vi "RDS Child Receive Message.vi"(8 "error in (no error)":errorcluster, 10 "RDS Message":refnum<class "RDS Message.lvclass">, 11 "AIP Instrument in":refnum<class "AIP Instrument.lvclass">) -> (0 "error out":errorcluster, 3 "AIP Instrument out":refnum<class "AIP Instrument.lvclass">)   [LabVIEW 2015, in "AIP Instrument.lvlib" / "AIP Instrument.lvclass"]
uses:
  AIP Instrument.lvclass
  Libraries/RDS Framework/RDS Message Class/RDS Message.lvclass
  Libraries/RDS Framework/RDS Message Class/RDS Message.lvclass/RDS Message.ctl
  Libraries/RDS Framework/RDS Message Class/AIP Command.lvclass
  Libraries/RDS Framework/RDS Message Class/AIP Command.lvclass/AIP Command.ctl
  Libraries/RDS Serial Handler/RDS Serial Frame.lvclass/RDS Serial Frame.ctl
  AIP Instrument.lvclass/AIP Instrument.ctl
  Libraries/RDS Child Messages/Depth Data Message/Depth Data Message.lvclass
  Libraries/RDS Instruments/AIP/AIP Status.ctl
  Libraries/RDS Instruments/AIP/AIP States.ctl
  Libraries/RDS Child Messages/Depth Data Message/Depth Data Message.lvclass/Depth Data Message.ctl
  Libraries/RDS Child Messages/AIP Set Min Depth Message/AIP Set Min Depth Message.lvclass
  Libraries/RDS Child Messages/AIP Set Min Depth Message/AIP Set Min Depth Message.lvclass/AIP Set Min Depth Message.ctl
  Libraries/RDS Serial Handler/RDS Serial Frame.lvclass
  Actors/RDS Serial Instrument Actor/RDS Serial Instrument Actor.lvclass
  Libraries/RDS Instruments/RDS Instrument Library.lvlib
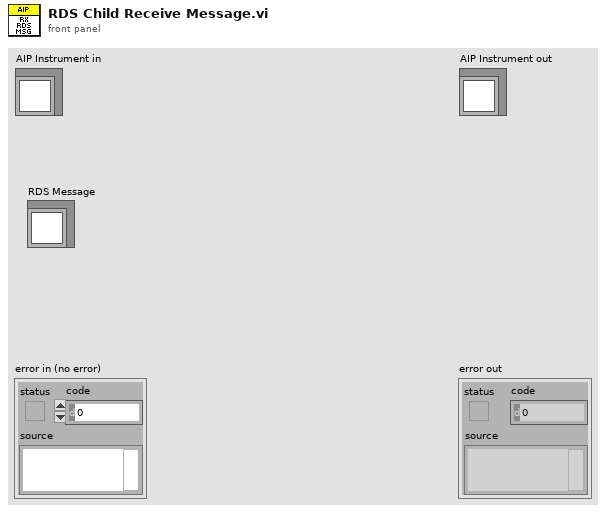
[diagram p1: front panel]
types:
  T1 = typedef "RDS Child Messages.lvlib/RDS Message ID.ctl" = enum16{"RDS Hello World", "String Message", "AIP_Status", "AIP_Command", "GPS_Data", "MCB_Command", "MCB_Status", "Compass_Data", "Depth_Data", "Battery_Data", "Contoller_State", "Set_Mag_Dev", "BTB_Shutdown", "State_Sample_Request", "State_Sample", "PID_Gains_Set", "Helm_Limiter_Set", "Helm_Heading_Command", "Helm_Steering_Command", "Helm_Status", "Controller_Message", "AIP_Set_Min_Depth", "Mission_Controller_State", "Mission_Upload", "Mission_Set_Op_and_Run", "Mission_Settings_Set"}
  T2 = typedef "RDS Instrument Library.lvlib/AIP Status.ctl" = cluster{"FWD Port":T3, "FWD Stbd":T3, "AFT Port":T3, "AFT Stbd":T3, "AIP Depth Min":u8}
  T3 = typedef "RDS Instrument Library.lvlib/AIP States.ctl" = enum16{"Deploy", "Deploying", "Deployed", "Stow", "Stowing", "Stowed", "Fault", "brakeOnStow", "breakOnDeploy", "Stopped", "Stopping"}
  T4 = typedef "RDS Child Messages.lvlib/AIP Command Control.ctl" = enum16{"Stow", "Deploy", "Stop", "Validate Sensors", "Jog Deploy FP", "Jog Stow FP", "Jog Deploy FS", "Jog Stow FS", "Jog Deploy AP", "Jog Stow AP", "Jog Deploy AS", "Jog Stow AS", "Deploy FP", "Deploy FS", "Deploy AP", "Deploy AS", "Stow FP", "Stow FS", "Stow AP", "Stow AS"}
  T5 = typedef "RDS Child Messages.lvlib/Depth Data.ctl" = cluster{"Depth":sgl, "Water Temp":i8}
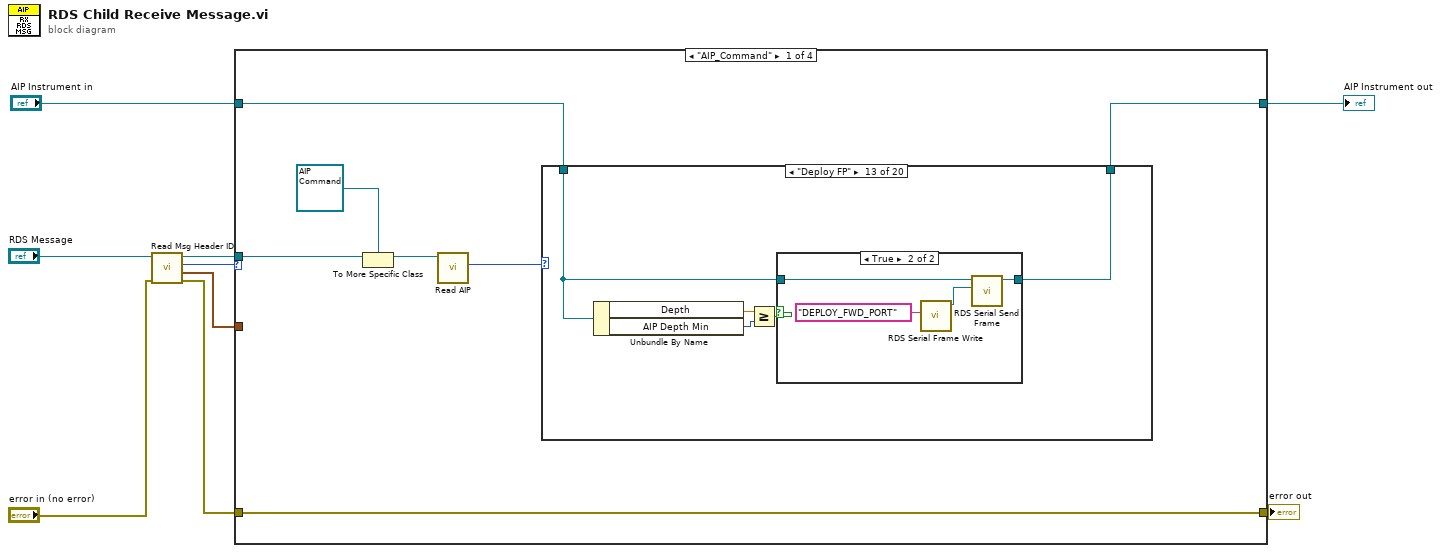
[diagram p0: block diagram]
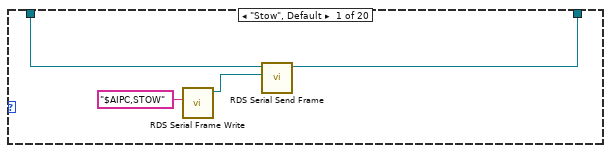
[diagram p2: hidden frame]
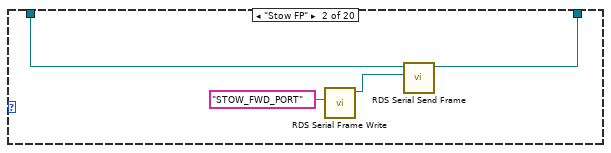
[diagram p3: hidden frame]
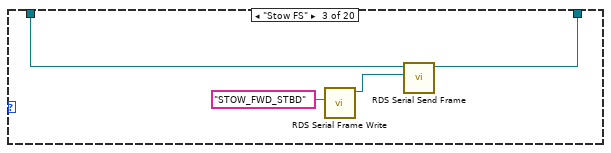
[diagram p4: hidden frame]
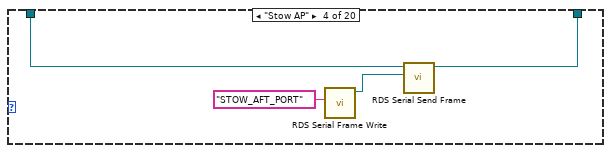
[diagram p5: hidden frame]
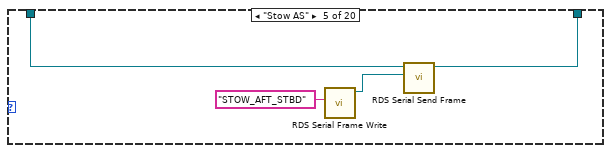
[diagram p6: hidden frame]
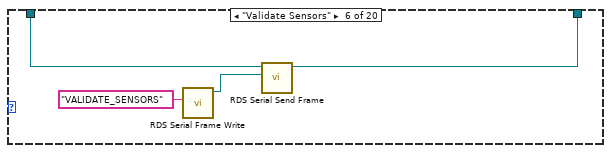
[diagram p7: hidden frame]
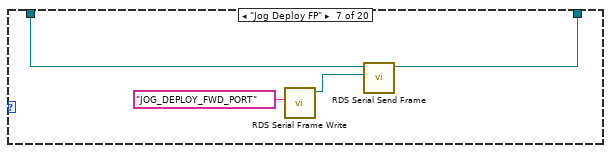
[diagram p8: hidden frame]
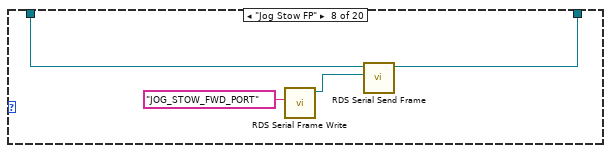
[diagram p9: hidden frame]
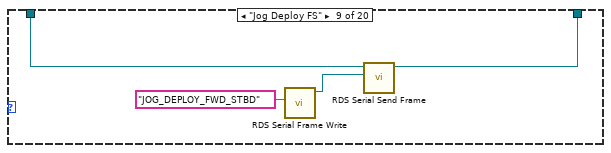
[diagram p10: hidden frame]
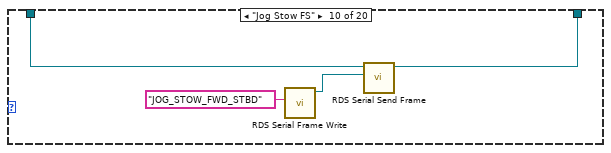
[diagram p11: hidden frame]
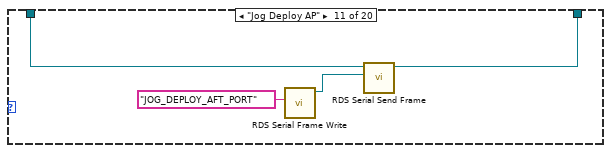
[diagram p12: hidden frame]
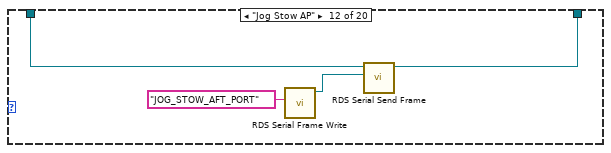
[diagram p13: hidden frame]
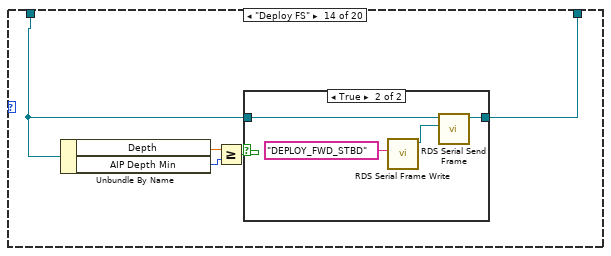
[diagram p15: hidden frame]
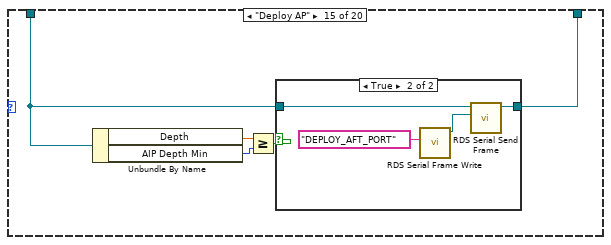
[diagram p17: hidden frame]
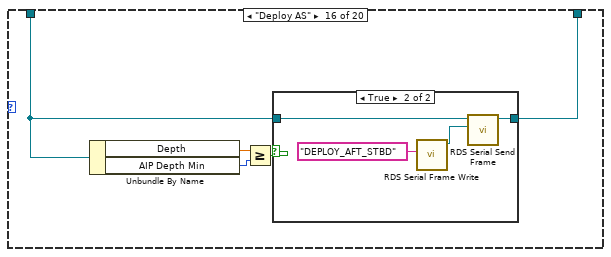
[diagram p19: hidden frame]
diagram:
  n1 = call "Read Msg Header ID.vi"("error in (no error)"="error in (no error)", "RDS Message in"="RDS Message") -> ("error out"=w6:errorcluster, "Time Stamp"=w7:timestamp, "Msg ID"=w9:T1, "RDS Message out"=w8:refnum<class "RDS Message.lvclass">)  [unwired: 5 in, 1 out]
  n2 = case shown="\"AIP_Command\"" w9 {
    tunnel: "AIP Instrument in" -> [w11 w128 w138 w152]
    tunnel: w8 -> [w14 _ w142 w156]
    tunnel: [w10 w128 w129 w151] -> w2
    tunnel: w7 -> [_ _ _ _]
    tunnel: w6 -> [w16 w127 w144 w157]
    tunnel: [w16 w127 w144 w157] -> w1
    frame "AIP_Command" {
      n3 = To More Specific Class(target class=refnum<class "AIP Command.lvclass"> refnum ("RDS Child Messages.lvlib:AIP Command.lvclass"), reference=w14) -> (specific class reference=w13:refnum<class "AIP Command.lvclass">)  [unwired: 1 in, 1 out]
      n4 = call "Read AIP.vi"("AIP Deploy Command in"=w13) -> ("AIP Command"=w12:T4)  [unwired: 8 in, 2 out]
      n5 = case shown="\"Deploy FP\"" w12 {
        tunnel: w11 -> [w18 w22 w26 w30 w34 w38 w42 w46 w50 w54 w58 w62 w66 w76 w86 w95 w106 w110 w116 w126]
        tunnel: [w17 w21 w25 w29 w33 w37 w41 w45 w49 w53 w57 w61 w65 w75 w85 w96 w105 w109 w117 w123] -> w10
        frame "Stow", Default {
          n6 = call "RDS Serial Frame Write.vi"("Serial String"="$AIPC,STOW") -> ("RDS Serial Frame out"=w19:refnum<class "RDS Serial Frame.lvclass">)  [unwired: 9 in, 1 out]
          n7 = call "RDS Serial Send Frame.vi"("RDS Frame"=w19, "RDS Serial Instrument Actor in"=w18) -> ("RDS Serial Instrument Actor out"=w17:refnum<class "AIP Instrument.lvclass">)  [unwired: 8 in, 1 out]
        }
        frame "Stow FP" {
          n8 = call "RDS Serial Frame Write.vi"("Serial String"="STOW_FWD_PORT") -> ("RDS Serial Frame out"=w23:refnum<class "RDS Serial Frame.lvclass">)  [unwired: 9 in, 1 out]
          n9 = call "RDS Serial Send Frame.vi"("RDS Frame"=w23, "RDS Serial Instrument Actor in"=w22) -> ("RDS Serial Instrument Actor out"=w21:refnum<class "AIP Instrument.lvclass">)  [unwired: 8 in, 1 out]
        }
        frame "Stow FS" {
          n10 = call "RDS Serial Frame Write.vi"("Serial String"="STOW_FWD_STBD") -> ("RDS Serial Frame out"=w27:refnum<class "RDS Serial Frame.lvclass">)  [unwired: 9 in, 1 out]
          n11 = call "RDS Serial Send Frame.vi"("RDS Frame"=w27, "RDS Serial Instrument Actor in"=w26) -> ("RDS Serial Instrument Actor out"=w25:refnum<class "AIP Instrument.lvclass">)  [unwired: 8 in, 1 out]
        }
        frame "Stow AP" {
          n12 = call "RDS Serial Frame Write.vi"("Serial String"="STOW_AFT_PORT") -> ("RDS Serial Frame out"=w31:refnum<class "RDS Serial Frame.lvclass">)  [unwired: 9 in, 1 out]
          n13 = call "RDS Serial Send Frame.vi"("RDS Frame"=w31, "RDS Serial Instrument Actor in"=w30) -> ("RDS Serial Instrument Actor out"=w29:refnum<class "AIP Instrument.lvclass">)  [unwired: 8 in, 1 out]
        }
        frame "Stow AS" {
          n14 = call "RDS Serial Frame Write.vi"("Serial String"="STOW_AFT_STBD") -> ("RDS Serial Frame out"=w35:refnum<class "RDS Serial Frame.lvclass">)  [unwired: 9 in, 1 out]
          n15 = call "RDS Serial Send Frame.vi"("RDS Frame"=w35, "RDS Serial Instrument Actor in"=w34) -> ("RDS Serial Instrument Actor out"=w33:refnum<class "AIP Instrument.lvclass">)  [unwired: 8 in, 1 out]
        }
        frame "Validate Sensors" {
          n16 = call "RDS Serial Frame Write.vi"("Serial String"="VALIDATE_SENSORS") -> ("RDS Serial Frame out"=w39:refnum<class "RDS Serial Frame.lvclass">)  [unwired: 9 in, 1 out]
          n17 = call "RDS Serial Send Frame.vi"("RDS Frame"=w39, "RDS Serial Instrument Actor in"=w38) -> ("RDS Serial Instrument Actor out"=w37:refnum<class "AIP Instrument.lvclass">)  [unwired: 8 in, 1 out]
        }
        frame "Jog Deploy FP" {
          n18 = call "RDS Serial Frame Write.vi"("Serial String"="JOG_DEPLOY_FWD_PORT") -> ("RDS Serial Frame out"=w43:refnum<class "RDS Serial Frame.lvclass">)  [unwired: 9 in, 1 out]
          n19 = call "RDS Serial Send Frame.vi"("RDS Frame"=w43, "RDS Serial Instrument Actor in"=w42) -> ("RDS Serial Instrument Actor out"=w41:refnum<class "AIP Instrument.lvclass">)  [unwired: 8 in, 1 out]
        }
        frame "Jog Stow FP" {
          n20 = call "RDS Serial Frame Write.vi"("Serial String"="JOG_STOW_FWD_PORT") -> ("RDS Serial Frame out"=w47:refnum<class "RDS Serial Frame.lvclass">)  [unwired: 9 in, 1 out]
          n21 = call "RDS Serial Send Frame.vi"("RDS Frame"=w47, "RDS Serial Instrument Actor in"=w46) -> ("RDS Serial Instrument Actor out"=w45:refnum<class "AIP Instrument.lvclass">)  [unwired: 8 in, 1 out]
        }
        frame "Jog Deploy FS" {
          n22 = call "RDS Serial Frame Write.vi"("Serial String"="JOG_DEPLOY_FWD_STBD") -> ("RDS Serial Frame out"=w51:refnum<class "RDS Serial Frame.lvclass">)  [unwired: 9 in, 1 out]
          n23 = call "RDS Serial Send Frame.vi"("RDS Frame"=w51, "RDS Serial Instrument Actor in"=w50) -> ("RDS Serial Instrument Actor out"=w49:refnum<class "AIP Instrument.lvclass">)  [unwired: 8 in, 1 out]
        }
        frame "Jog Stow FS" {
          n24 = call "RDS Serial Frame Write.vi"("Serial String"="JOG_STOW_FWD_STBD") -> ("RDS Serial Frame out"=w55:refnum<class "RDS Serial Frame.lvclass">)  [unwired: 9 in, 1 out]
          n25 = call "RDS Serial Send Frame.vi"("RDS Frame"=w55, "RDS Serial Instrument Actor in"=w54) -> ("RDS Serial Instrument Actor out"=w53:refnum<class "AIP Instrument.lvclass">)  [unwired: 8 in, 1 out]
        }
        frame "Jog Deploy AP" {
          n26 = call "RDS Serial Frame Write.vi"("Serial String"="JOG_DEPLOY_AFT_PORT") -> ("RDS Serial Frame out"=w59:refnum<class "RDS Serial Frame.lvclass">)  [unwired: 9 in, 1 out]
          n27 = call "RDS Serial Send Frame.vi"("RDS Frame"=w59, "RDS Serial Instrument Actor in"=w58) -> ("RDS Serial Instrument Actor out"=w57:refnum<class "AIP Instrument.lvclass">)  [unwired: 8 in, 1 out]
        }
        frame "Jog Stow AP" {
          n28 = call "RDS Serial Frame Write.vi"("Serial String"="JOG_STOW_AFT_PORT") -> ("RDS Serial Frame out"=w63:refnum<class "RDS Serial Frame.lvclass">)  [unwired: 9 in, 1 out]
          n29 = call "RDS Serial Send Frame.vi"("RDS Frame"=w63, "RDS Serial Instrument Actor in"=w62) -> ("RDS Serial Instrument Actor out"=w61:refnum<class "AIP Instrument.lvclass">)  [unwired: 8 in, 1 out]
        }
        frame "Deploy FP" {
          n30 = Unbundle By Name(w66) -> ("Depth"=w68:sgl, "AIP Depth Min"=w67:u8)
          n31 = Greater Or Equal?(x=w68, y=w67) -> (x >= y?=w69:bool)
          n32 = case shown="True" w69 {
            tunnel: [w70 w72] -> w65
            tunnel: w66 -> [w70 w71]
            frame False {
              # "TOO SHALLOW!"
            }
            frame True {
              n33 = call "RDS Serial Frame Write.vi"("Serial String"="DEPLOY_FWD_PORT") -> ("RDS Serial Frame out"=w73:refnum<class "RDS Serial Frame.lvclass">)  [unwired: 9 in, 1 out]
              n34 = call "RDS Serial Send Frame.vi"("RDS Frame"=w73, "RDS Serial Instrument Actor in"=w71) -> ("RDS Serial Instrument Actor out"=w72:refnum<class "AIP Instrument.lvclass">)  [unwired: 8 in, 1 out]
            }
          }
        }
        frame "Deploy FS" {
          n35 = Unbundle By Name(w76) -> ("Depth"=w78:sgl, "AIP Depth Min"=w77:u8)
          n36 = Greater Or Equal?(x=w78, y=w77) -> (x >= y?=w79:bool)
          n37 = case shown="True" w79 {
            tunnel: [w80 w82] -> w75
            tunnel: w76 -> [w80 w81]
            frame False {
              # "TOO SHALLOW!"
            }
            frame True {
              n38 = call "RDS Serial Frame Write.vi"("Serial String"="DEPLOY_FWD_STBD") -> ("RDS Serial Frame out"=w83:refnum<class "RDS Serial Frame.lvclass">)  [unwired: 9 in, 1 out]
              n39 = call "RDS Serial Send Frame.vi"("RDS Frame"=w83, "RDS Serial Instrument Actor in"=w81) -> ("RDS Serial Instrument Actor out"=w82:refnum<class "AIP Instrument.lvclass">)  [unwired: 8 in, 1 out]
            }
          }
        }
        frame "Deploy AP" {
          n40 = Unbundle By Name(w86) -> ("Depth"=w88:sgl, "AIP Depth Min"=w87:u8)
          n41 = Greater Or Equal?(x=w88, y=w87) -> (x >= y?=w89:bool)
          n42 = case shown="True" w89 {
            tunnel: [w90 w92] -> w85
            tunnel: w86 -> [w90 w91]
            frame False {
              # "TOO SHALLOW!"
            }
            frame True {
              n43 = call "RDS Serial Frame Write.vi"("Serial String"="DEPLOY_AFT_PORT") -> ("RDS Serial Frame out"=w93:refnum<class "RDS Serial Frame.lvclass">)  [unwired: 9 in, 1 out]
              n44 = call "RDS Serial Send Frame.vi"("RDS Frame"=w93, "RDS Serial Instrument Actor in"=w91) -> ("RDS Serial Instrument Actor out"=w92:refnum<class "AIP Instrument.lvclass">)  [unwired: 8 in, 1 out]
            }
          }
        }
        frame "Deploy AS" {
          n45 = Unbundle By Name(w95) -> ("Depth"=w98:sgl, "AIP Depth Min"=w97:u8)
          n46 = Greater Or Equal?(x=w98, y=w97) -> (x >= y?=w99:bool)
          n47 = case shown="True" w99 {
            tunnel: [w100 w102] -> w96
            tunnel: w95 -> [w100 w101]
            frame False {
              # "TOO SHALLOW!"
            }
            frame True {
              n48 = call "RDS Serial Frame Write.vi"("Serial String"="DEPLOY_AFT_STBD") -> ("RDS Serial Frame out"=w103:refnum<class "RDS Serial Frame.lvclass">)  [unwired: 9 in, 1 out]
              n49 = call "RDS Serial Send Frame.vi"("RDS Frame"=w103, "RDS Serial Instrument Actor in"=w101) -> ("RDS Serial Instrument Actor out"=w102:refnum<class "AIP Instrument.lvclass">)  [unwired: 8 in, 1 out]
            }
          }
        }
        frame "Jog Deploy AS" {
          n50 = call "RDS Serial Frame Write.vi"("Serial String"="JOG_DEPLOY_AFT_STBD") -> ("RDS Serial Frame out"=w107:refnum<class "RDS Serial Frame.lvclass">)  [unwired: 9 in, 1 out]
          n51 = call "RDS Serial Send Frame.vi"("RDS Frame"=w107, "RDS Serial Instrument Actor in"=w106) -> ("RDS Serial Instrument Actor out"=w105:refnum<class "AIP Instrument.lvclass">)  [unwired: 8 in, 1 out]
        }
        frame "Jog Stow AS" {
          n52 = call "RDS Serial Frame Write.vi"("Serial String"="JOG_STOW_AFT_STBD") -> ("RDS Serial Frame out"=w111:refnum<class "RDS Serial Frame.lvclass">)  [unwired: 9 in, 1 out]
          n53 = call "RDS Serial Send Frame.vi"("RDS Frame"=w111, "RDS Serial Instrument Actor in"=w110) -> ("RDS Serial Instrument Actor out"=w109:refnum<class "AIP Instrument.lvclass">)  [unwired: 8 in, 1 out]
        }
        frame "Deploy" {
          n54 = Unbundle By Name(w116) -> ("Depth"=w114:sgl, "AIP Depth Min"=w113:u8)
          n55 = Greater Or Equal?(x=w114, y=w113) -> (x >= y?=w115:bool)
          n56 = case shown="True" w115 {
            tunnel: [w118 w120] -> w117
            tunnel: w116 -> [w118 w119]
            frame False {
              # "TOO SHALLOW!"
            }
            frame True {
              n57 = call "RDS Serial Frame Write.vi"("Serial String"="$AIPC,DEPLOY") -> ("RDS Serial Frame out"=w121:refnum<class "RDS Serial Frame.lvclass">)  [unwired: 9 in, 1 out]
              n58 = call "RDS Serial Send Frame.vi"("RDS Frame"=w121, "RDS Serial Instrument Actor in"=w119) -> ("RDS Serial Instrument Actor out"=w120:refnum<class "AIP Instrument.lvclass">)  [unwired: 8 in, 1 out]
            }
          }
        }
        frame "Stop" {
          n59 = call "RDS Serial Frame Write.vi"("Serial String"="$AIPC,STOP") -> ("RDS Serial Frame out"=w124:refnum<class "RDS Serial Frame.lvclass">)  [unwired: 9 in, 1 out]
          n60 = call "RDS Serial Send Frame.vi"("RDS Frame"=w124, "RDS Serial Instrument Actor in"=w126) -> ("RDS Serial Instrument Actor out"=w123:refnum<class "AIP Instrument.lvclass">)  [unwired: 8 in, 1 out]
        }
      }
    }
    frame "String Message", Default {
    }
    frame "Depth_Data" {
      n61 = To More Specific Class(target class=refnum<class "Depth Data Message.lvclass"> refnum ("RDS Child Messages.lvlib:Depth Data Message.lvclass"), reference=w142) -> (specific class reference=w141:refnum<class "Depth Data Message.lvclass">)  [unwired: 1 in, 1 out]
      n62 = call "Read Depth Data.vi"("Depth Data Message in"=w141) -> ("Depth Data"=w140:T5)  [unwired: 8 in, 2 out]
      n63 = Unbundle By Name(w140) -> ("Depth"=w139:sgl)
      n64 = Bundle By Name(cluster=w138, "Depth"=w139) -> (w130:refnum<class "AIP Instrument.lvclass">)
      n65 = Unbundle By Name(w130) -> ("AIP State"=w135:T2, "Depth"=w137:sgl, "AIP Depth Min"=w136:u8)
      n66 = Not Equal?(x=T2 {"FWD Port"=enum."Stowed", "FWD Stbd"=enum."Stowed", "AFT Port"=enum."Stowed", "AFT Stbd"=enum."Stowed", "AIP Depth Min"=0}, y=w135) -> (x != y?=w133:bool)
      n67 = Less?(x=w137, y=w136) -> (x < y?=w132:bool)
      n68 = And(x=w133, y=w132) -> (x .and. y?=w131:bool)
      n69 = case shown="False" w131 {
        tunnel: w130 -> [w145 w148]
        tunnel: [w145 w147] -> w129
        frame False {
        }
        frame True {
          n70 = call "RDS Serial Frame Write.vi"("Serial String"="$AIPC,STOW") -> ("RDS Serial Frame out"=w149:refnum<class "RDS Serial Frame.lvclass">)  [unwired: 9 in, 1 out]
          n71 = Wait (ms)(milliseconds to wait=u32 1000) -> ()  [unwired: 1 out]
          n72 = call "RDS Serial Send Frame.vi"("RDS Frame"=w149, "RDS Serial Instrument Actor in"=w148) -> ("RDS Serial Instrument Actor out"=w147:refnum<class "AIP Instrument.lvclass">)  [unwired: 8 in, 1 out]
        }
      }
    }
    frame "AIP_Set_Min_Depth" {
      n73 = To More Specific Class(target class=refnum<class "AIP Set Min Depth Message.lvclass"> refnum ("RDS Child Messages.lvlib:AIP Set Min Depth Message.lvclass"), reference=w156) -> (specific class reference=w154:refnum<class "AIP Set Min Depth Message.lvclass">)  [unwired: 1 in, 1 out]
      n74 = call "Read Min Depth Message.vi"("AIP Set Min Depth Message in"=w154) -> ("Min Depth"=w153:u8)  [unwired: 8 in, 2 out]
      n75 = Bundle By Name(cluster=w152, "AIP Depth Min"=w153) -> (w151:refnum<class "AIP Instrument.lvclass">)
    }
  }
  "error out" <- w1
  "AIP Instrument out" <- w2
